vi "NADC Sync Out.vi"(5 "Rate (T:FULL)":bool=TRUE, 7 "Begin Timeslot (1)":i16=1, 8 "error in (no error)":errorcluster {"code" format="%.0x"}, 9 "Sync Out Offset (0)":i16, 10 "Sync Out (0:BEGIN FRAME)":T1(ring), 11 "VISA Resource Name":refnum<visa-resource-name>) -> (0 "error out":errorcluster {"code" format="%.0x"}, 3 "VISA Resource Name Out":refnum<visa-resource-name>)   [LabVIEW 2014, in "Agilent ESG Series.lvlib"]
doc: "This VI is used to configure the \"Sync Out\" parameters.\nThere is no need to run this vi if Data Format is set to Pattern because the Sync out will default to Begin Pattern."
uses:
  Agilent ESG Series.lvlib
panel:
  # "FULL"
  # "HALF"
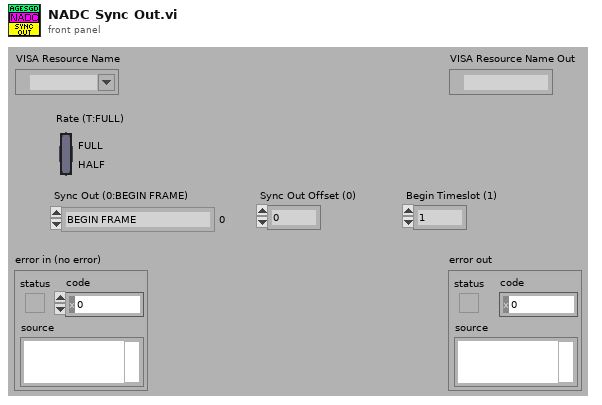
[diagram p1: front panel]
types:
  T1 = enum16{"BEGIN FRAME", "BEGIN TIMESLOT", "ALL TIMESLOTS"}
  T2 = cluster{"status":bool, "code":i32, "VI Name":string}
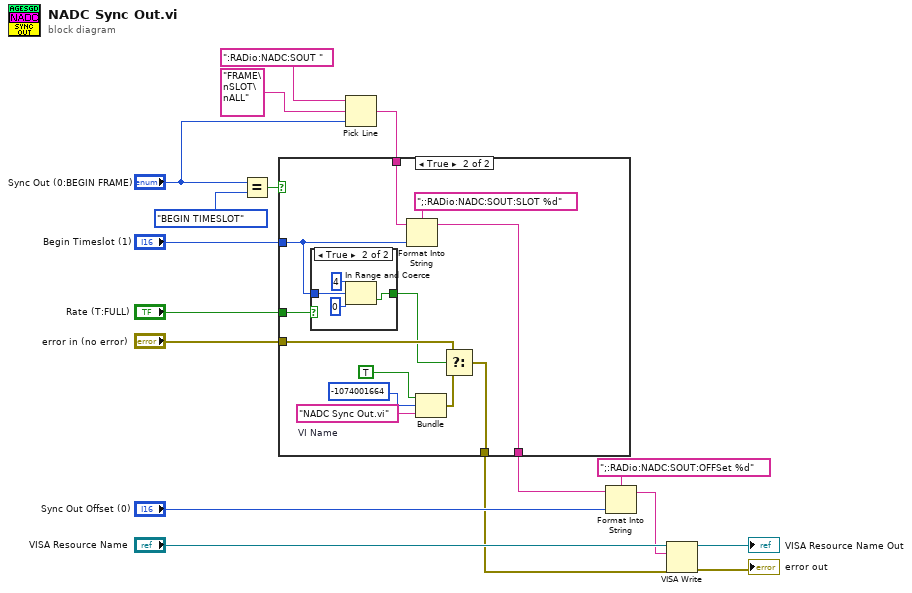
[diagram p0: block diagram]
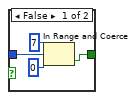
[diagram p3: hidden frame]
diagram:
  n1 = Equal?(x="Sync Out (0:BEGIN FRAME)", y=T1."BEGIN TIMESLOT") -> (x = y?=w3:bool)
  n2 = Pick Line(string ("")=":RADio:NADC:SOUT ", multi-line string="FRAME\nSLOT\nALL", line index="Sync Out (0:BEGIN FRAME)") -> (output string=w11:string)
  n3 = case shown="True" w3 {
    tunnel: "Begin Timeslot (1)" -> [_ w21]
    tunnel: w11 -> [w19 w20]
    tunnel: [w19 w30] -> w2
    tunnel: "Rate (T:FULL)" -> [_ w29]
    tunnel: "error in (no error)" -> [w18 w25]
    tunnel: [w18 w24] -> w8
    frame False {
    }
    frame True {
      w28 = "NADC Sync Out.vi"  # VI Name
      n4 = case shown="True" w29 {
        tunnel: [w35 w39] -> w22
        tunnel: w21 -> [w34 w38]
        frame False {
          n5 = In Range and Coerce(upper limit=i16 7 ("hi"), x=w34, lower limit=i16 0 ("lo")) -> (In Range?=w35:bool)  [unwired: 1 out]
        }
        frame True {
          n6 = In Range and Coerce(upper limit=i16 4 ("hi"), x=w38, lower limit=i16 0 ("lo")) -> (In Range?=w39:bool)  [unwired: 1 out]
        }
      }
      n7 = Format Into String(format string=";:RADio:NADC:SOUT:SLOT %d", initial string=w20, w21) -> (resulting string=w30:string)  [unwired: 1 in, 1 out]
      n8 = Bundle(TRUE, -1074001664, "VI Name"=w28) -> (w23:cluster{bool, i32, "VI Name":string})  [unwired: 1 in]
      n9 = Select(t=w25, s=w22, f=w23) -> (s? t:f=w24:T2)
    }
  }
  n10 = Format Into String(format string=";:RADio:NADC:SOUT:OFFSet %d", initial string=w2, "Sync Out Offset (0)") -> (resulting string=w7:string)  [unwired: 1 in, 1 out]
  n11 = VISA Write(VISA resource name="VISA Resource Name", write buffer=w7, error in (no error)=w8) -> (VISA resource name out=→"VISA Resource Name Out":refnum<visa-resource-name>, error out=→"error out":errorcluster)  [unwired: 1 out]
